vi "run.json_to_object.vi"(8 "error in":errorcluster, 11 "JSON":string) -> (0 "error out":errorcluster, 2 "Run":refnum<class "Run.lvclass">)   [LabVIEW 2020, in "Nominal Client.lvclass"]
uses:
  Nominal Client.lvclass
  Run/Run.lvclass
  a6937c0b-1e56-4696-aef8-7c551fe44323.vi
  <vilib>/JDP Science/JSONtext/JSON text to Variant.vi
  <vilib>/JDP Science/JSONtext/LVClass Serializer/JSONtext LVClass Serializer.lvclass
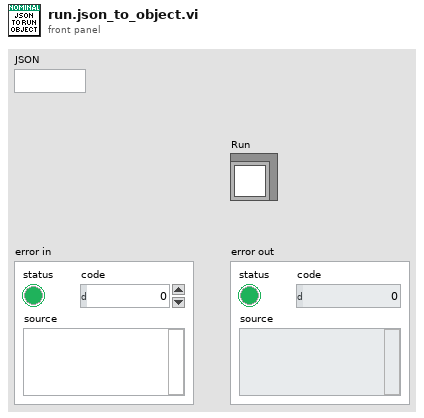
[diagram p1: front panel]
types:
  T1 = cluster{"rid":string, "runNumber":i32, "title":string, "description":string, "startTime":cluster{"secondsSinceEpoch":i32, "offsetNanoseconds":i32}, "properties":map{string, cluster{"url":string, "title":string}[]}, "labels":string[], "links":cluster{"url":string, "title":string}[], "createdAt":string, "updatedAt":string, "attachments":string[], "assets":string[], "runPrefix":string, "authorRid":string, "endTime":cluster{"secondsSinceEpoch":i32, "offsetNanoseconds":i32}, "asset":string}
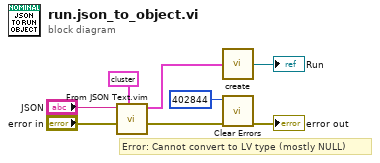
[diagram p0: block diagram]
diagram:
  # "Error: Cannot convert to LV type (mostly NULL)"
  n1 = call "From JSON Text.vim"("Data Type and Default Value"=T1 {"rid"="", "runNumber"=0, "title"="", "description"="", "startTime"={"secondsSinceEpoch"=0, "offsetNanoseconds"=0}, "properties"={}, "labels"=[], "links"=[], "createdAt"="", "updatedAt"="", "attachments"=[], "assets"=[], "runPrefix"="", "authorRid"="", "endTime"={"secondsSinceEpoch"=0, "offsetNanoseconds"=0}, "asset"=""} ("Response"), "error in (no error)"="error in", "JSON"="JSON") -> ("error out"=w7:errorcluster, "Data out"=w5:T1)  [unwired: 7 in]
  n2 = call "create.vi"("Run Data"=w5) -> ("Run"=→"Run":refnum<class "Run.lvclass">)
  n3 = call <vilib>:"Clear Errors.vi"("error in (no error)"=w7, "specific error code to clear (0: all)"=402844) -> ("error out"=→"error out":errorcluster)  [unwired: 4 in, 1 out]
